vi "Create Spreadsheet Header.vi"(10 "Channel Settings":T1[](array[typedef])) -> (2 "Log file header":string)   [LabVIEW 2021, in "Logging.lvlib"]
uses:
  Logging.lvlib
  Acquisition/Channel Settings.ctl
  Acquisition/IO Device.ctl
  Acquisition/Acquisition.lvlib
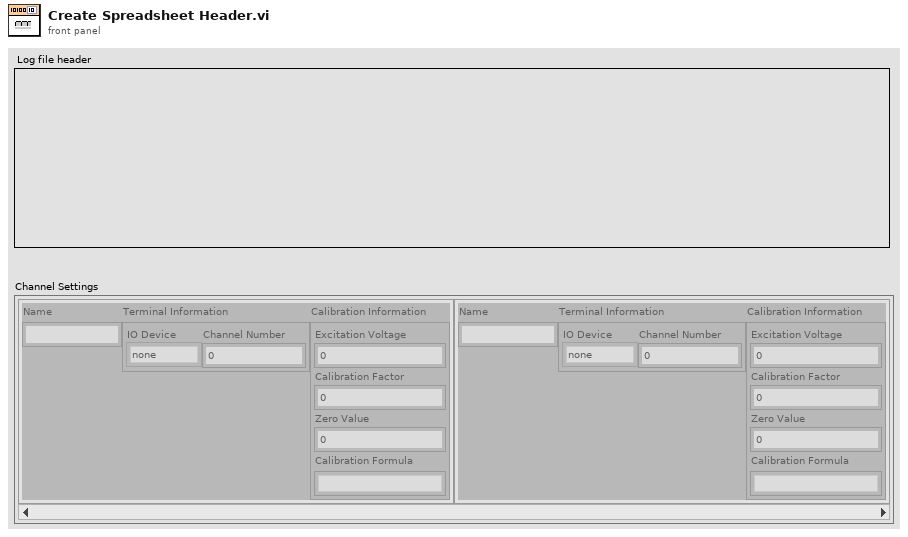
[diagram p1: front panel]
types:
  T1 = typedef "Acquisition.lvlib/Channel Settings.ctl" = cluster{"Name":string, "Terminal Information":cluster{"IO Device":T2, "Channel Number":i32}, "Calibration Information":cluster{"Excitation Voltage":dbl, "Calibration Factor":dbl, "Zero Value":dbl, "Calibration Formula":string}}
  T2 = typedef "Acquisition.lvlib/IO Device.ctl" = enum16{"none", "9219", "9401"}
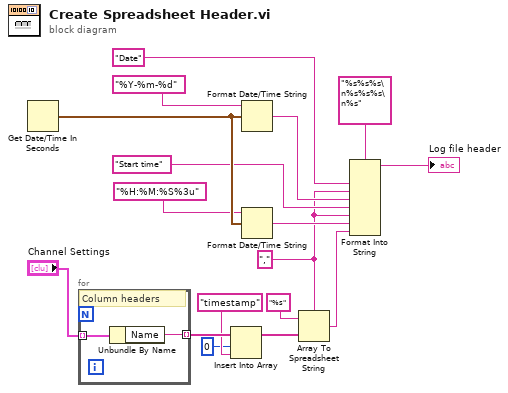
[diagram p0: block diagram]
diagram:
  w5 = "," ("delimiter (Tab)")
  n1 = Get Date/Time In Seconds() -> (seconds since 1Jan1904=w16:timestamp)
  n2 = for {
    tunnel: "Channel Settings" -> [w19] mode=indexing
    tunnel: [w18] -> w4 mode=indexing
    # "Column headers"
    n3 = Unbundle By Name(w19) -> ("Name"=w18:string)
  }
  n4 = Insert Into Array(array=w4, index=0, new element="timestamp" ("new element/subarray")) -> (w3:string[])
  n5 = Format Date/Time String(time format string (%c)="%Y-%m-%d", seconds (now)=w16) -> (date/time string=w12:string)  [unwired: 1 in]
  n6 = Format Date/Time String(time format string (%c)="%H:%M:%S%3u", seconds (now)=w16) -> (date/time string=w9:string)  [unwired: 1 in]
  n7 = Array To Spreadsheet String(delimiter (Tab)=w5, array=w3, 3:"%s" ("format string")) -> (spreadsheet string=w6:string)
  n8 = Format Into String(format string="%s%s%s\n%s%s%s\n%s", "Date", w5, w12, "Start time", w5, w9, w6) -> (resulting string=→"Log file header":string)  [unwired: 2 in, 1 out]
